vi "LoadRunCount.vi"(8 "error in":errorcluster, 10 "file path":path, 11 "APU Select":T1) -> (0 "error out":errorcluster, 3 "APURunCount":u32)   [LabVIEW 2018]
uses:
  Controller (Host)/Public Controls/APU Select.ctl
  <vilib>/Utility/config.llb/Read Key (U32).vi
  <vilib>/Utility/config.llb/NI_LVConfig.lvlib
  Controller (Host)/Controller (Host).lvlib
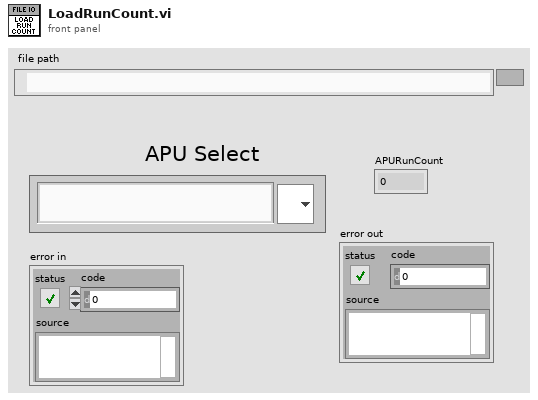
[diagram p1: front panel]
types:
  T1 = typedef "Controller (Host).lvlib/APU Select.ctl" = string
  T2 = typedef "NI_LVConfig.lvlib/Config Data RefNum.ctl" = refnum<k1>
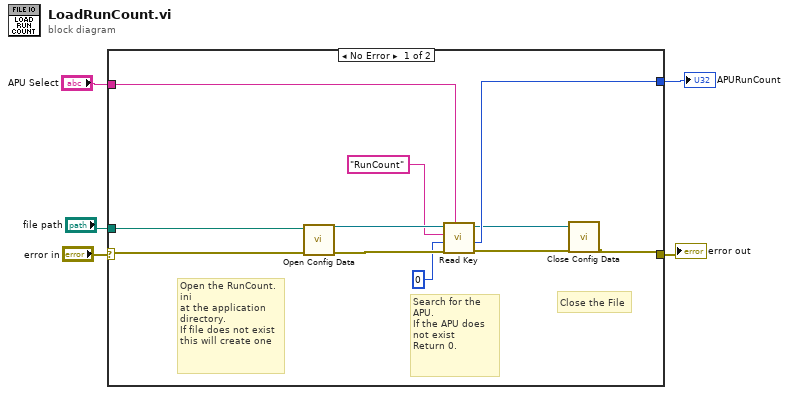
[diagram p0: block diagram]
diagram:
  n1 = case shown="No Error" "error in" {
    selector: "error in" -> [w16 w17]
    tunnel: "APU Select" -> [w8 _]
    tunnel: [w9 w17] -> w4
    tunnel: [w14 _] -> w5
    tunnel: "file path" -> [w6 _]
    frame No Error {
      # "Close the File"
      # "Search for the APU. \nIf the APU does not exist\nReturn 0."
      # "Open the RunCount.ini\nat the application directory. \nIf file does not exist this will create one"
      n2 = call <vilib>:"Open Config Data.vi"("error in (no error)"=w16, "configuration file path"=w6) -> ("error out"=w15:errorcluster, "refnum"=w13:T2)  [unwired: 7 in, 1 out]
      n3 = call-poly <vilib>:"Read Key.vi"("section"=w8, "error in (no error)"=w15, "default value"=u32 0, "key"="RunCount", "refnum"=w13) -> ("error out"=w10:errorcluster, "value"=w14:u32, "refnum out"=w11:T2)  [unwired: 3 in, 1 out]
      n4 = call <vilib>:"Close Config Data.vi"("error in (no error)"=w10, "refnum"=w11) -> ("error out"=w9:errorcluster)  [unwired: 8 in, 1 out]
    }
    frame Error {
    }
  }
  "APURunCount" <- w5
  "error out" <- w4
